vi "convertefreq.vi"(1 "Numeric":u16) -> (0 "string":string)   [LabVIEW 2019]
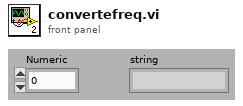
[diagram p1: front panel]
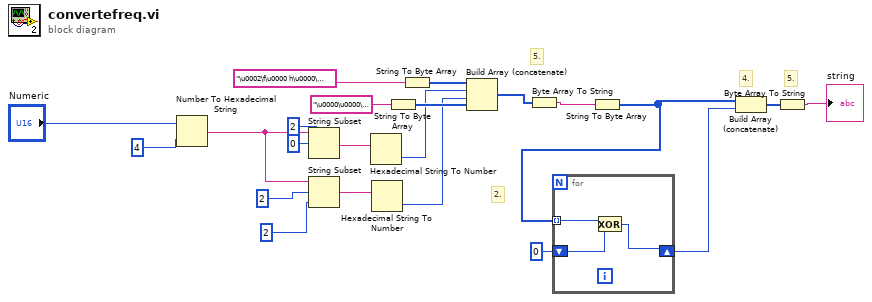
[diagram p0: block diagram]
diagram:
  # "5."
  # "4."
  # "2."
  # "5."
  n1 = Number To Hexadecimal String(1:i16 4 ("width (-)"), 2:"Numeric") -> (0:w13:string)
  n2 = String Subset(string=w13, offset (0)=0, length (rest)=2 ("length (rest)")) -> (substring=w12:string)
  n3 = String Subset(string=w13, offset (0)=2, length (rest)=2 ("length (rest)")) -> (substring=w10:string)
  n4 = Hexadecimal String To Number(string=w12) -> (number=w7:u32)  [unwired: 2 in, 1 out]
  n5 = Hexadecimal String To Number(string=w10) -> (number=w11:u32)  [unwired: 2 in, 1 out]
  n6 = String To Byte Array(string="\u0000\u0000\u0000\u0000" ("write buffer (\"\")")) -> (unsigned byte array=w21:u8[])
  n7 = String To Byte Array(string="\u0002\f\u0000 h\u0000\u0000" ("write buffer (\"\")")) -> (unsigned byte array=w3:u8[])
  n8 = Build Array (concatenate)(w3, w7, w11, w21) -> (w15:u32[])
  n9 = Byte Array To String(unsigned byte array=w15) -> (string=w16:string)
  n10 = String To Byte Array(string=w16) -> (unsigned byte array=w18:u8[])
  n11 = for {
    shift-right: [w24] -> w19
    shift-left: u8 0 -> [w25]
    tunnel: w18 -> [w23] mode=indexing
    n12 = Exclusive Or(1:w25, 2:w23) -> (0:w24:u8)
  }
  n13 = Build Array (concatenate)(w18, w19) -> (w17:u8[])
  n14 = Byte Array To String(unsigned byte array=w17) -> (string=→"string":string)
